vi "READ PLC FRAME.vi"(8 "errin":errorcluster, 10 "String in":string, 11 "Queue in":refnum<queue>) -> (0 "errout":errorcluster, 2 "String out":string, 3 "Queue out":refnum<queue>)   [LabVIEW 2020]
uses:
  VarGLO/Global PEAK.vi
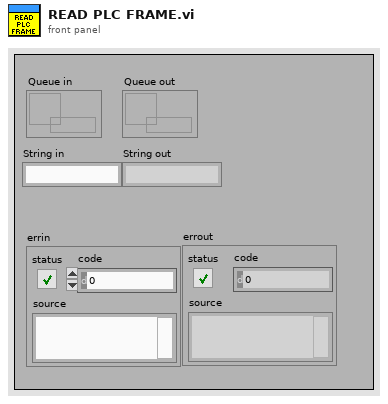
[diagram p1: front panel]
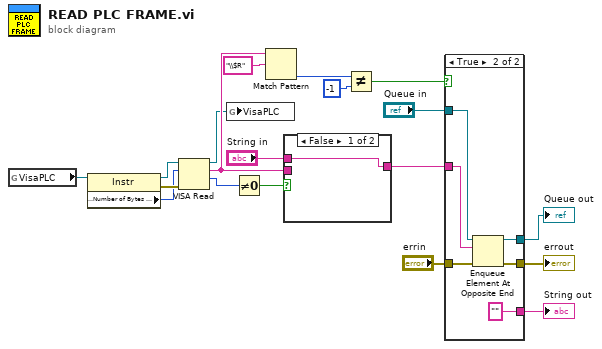
[diagram p0: block diagram]
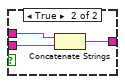
[diagram p2: hidden frame]
diagram:
  n1 = global read "Global PEAK.vi" "VisaPLC"() -> (w2:refnum<visa-resource-name>)
  n2 = property class="Instr"(reference=w2) -> (reference out=w12:refnum<visa-resource-name>, error out=w13:errorcluster, "Serial Settings:Number of Bytes at Serial Port"=w11:u32)  [unwired: 1 in]
  n3 = VISA Read(VISA resource name=w12, byte count=w11, error in (no error)=w13) -> (VISA resource name out=w1:refnum<visa-resource-name>, read buffer=w16:string, return count=w14:u32)  [unwired: 1 out]
  n4 = global write "Global PEAK.vi" "VisaPLC"(w1) -> ()
  n5 = Not Equal To 0?(x=w14) -> (x != 0?=w15:bool)
  n6 = Match Pattern ("Rechercher une expression")(string=w16, regular expression="\\$R" ("expression régulière")) -> (offset past match=w17:i32)  [unwired: 1 in, 3 out]
  n7 = case shown="False" w15 {
    tunnel: "String in" -> [w20 w23]
    tunnel: w16 -> [_ w22]
    tunnel: [w20 w21] -> w9
    frame False {
    }
    frame True {
      n8 = Concatenate Strings(w23, w22) -> (w21:string)
    }
  }
  n9 = Not Equal? ("Différents ?")(x=w17, y=-1) -> (x != y?=w4:bool)
  n10 = case shown="True" w4 {
    tunnel: "errin" -> [w25 w32]
    tunnel: [w25 w31] -> w6
    tunnel: "Queue in" -> [w26 w30]
    tunnel: [w26 w29] -> w8
    tunnel: w9 -> [w24 w28]
    tunnel: [w24 ""] -> w10
    frame False {
    }
    frame True {
      n11 = Enqueue Element At Opposite End(queue=w30, element=w28, error in (no error)=w32) -> (queue out=w29:refnum<queue>, error out=w31:errorcluster)  [unwired: 1 in, 1 out]
    }
  }
  "String out" <- w10
  "Queue out" <- w8
  "errout" <- w6
